vi "Shift Tag offsets for newly inserted data.vi"(4 "Litt/BigEnd":bool, 5 "Amount of data added\n(<0 means # of data bytesremoved)":i32, 6 "Ignore Tags":u16[](array[numeric]), 7 "error in":errorcluster, 8 "Byte stream offset\nwhere new data added":u32, 9 "Directories":T1[](array[typedef]), 10 "Image Data":u8[](array[numeric])) -> (0 "error out":errorcluster, 2 "Directories out":T1[](array[typedef]), 3 "Image Data Out":u8[](array[numeric]))   [LabVIEW 2013, in "Tiff reader.lvlib"]
doc: "This .vi shifts the tag Offsets for newly inserted data that might be inserted before the tags. or their pointer locations."
uses:
  Tiff reader.lvlib
  IFD Entry.ctl
  FieldTypes.ctl
  Word to bytes.vi
  Long word to bytes.vi
  Bytes to long word.vi
panel:
  out "Shifted?":bool
  out "Cluster":T1
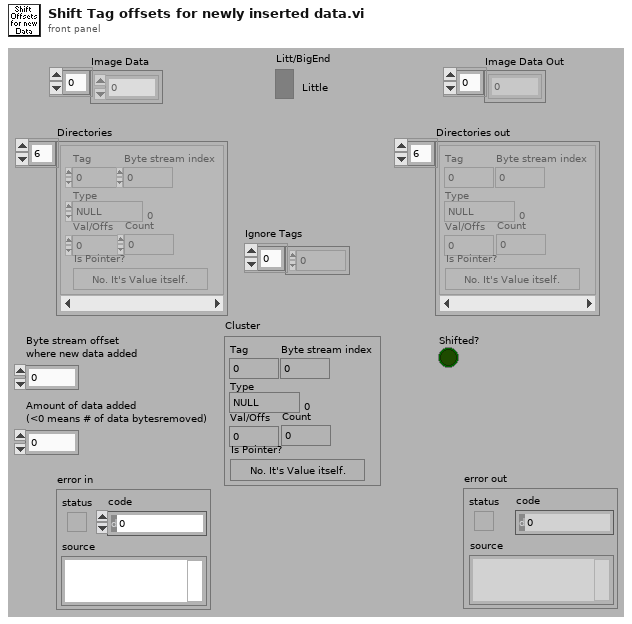
[diagram p1: front panel]
types:
  T1 = typedef "Tiff reader.lvlib/IFD Entry.ctl" = cluster{"Tag":u16, "Type":T2, "Count":u32, "Val/Offs":u32, "Is Pointer?":bool, "Byte stream index":i32}
  T2 = typedef "Tiff reader.lvlib/FieldTypes.ctl" = enum16{"NULL", "U8", "ASCII7", "U16", "U32", "RATIONAL", "SByte(I8)", "Undef(8Bit)", "I16", "I32", "SRat(4B:4B)", "SGL(4Byte)", "DBL(8Byte)"}
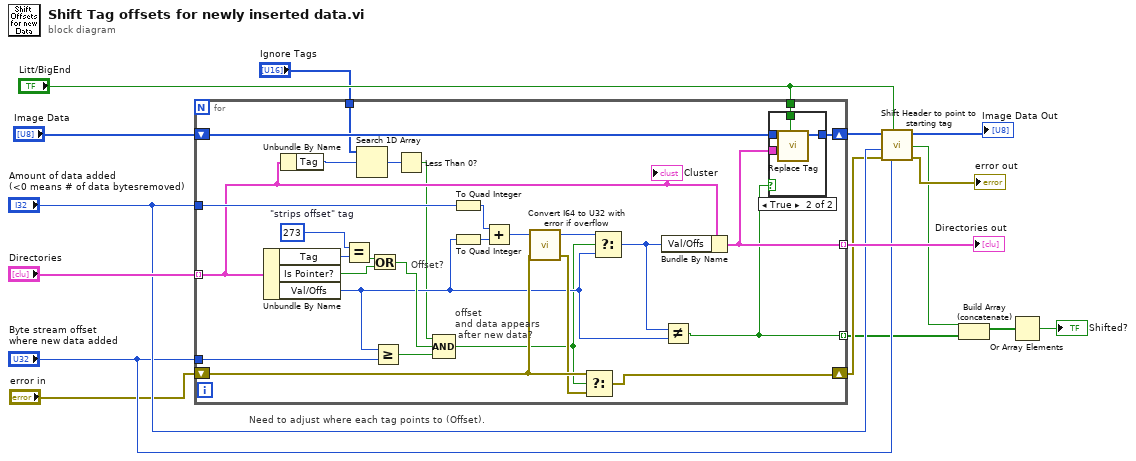
[diagram p0: block diagram]
diagram:
  # "Need to adjust where each tag points to (Offset)."
  n1 = for {
    tunnel: "Directories" -> [w20] mode=indexing
    tunnel: "Byte stream offset\nwhere new data added" -> [w42]
    tunnel: [w34] -> w15 mode=indexing
    tunnel: "Amount of data added\n(<0 means # of data bytesremoved)" -> [w39]
    tunnel: "Litt/BigEnd" -> [w37]
    shift-right: [w35] -> w13
    shift-left: "Image Data" -> [w36]
    shift-right: [w22] -> w8
    shift-left: "error in" -> [w44]
    tunnel: [w24] -> w4 mode=indexing
    tunnel: "Ignore Tags" -> [w21]
    w32 = u16 273  # "strips offset" tag
    # "Offset?"
    # "offset\nand data appears\n after new data?"
    n2 = Unbundle By Name(w20) -> ("Tag"=w33:u16, "Is Pointer?"=w30:bool, "Val/Offs"=w25:u32)
    n3 = Unbundle By Name(w20) -> ("Tag"=w19:u16)
    n4 = Equal?(x=w32, y=w33) -> (x = y?=w31:bool)
    n5 = Search 1D Array(1D array=w21, element=w19) -> (index of element=w18:i32)  [unwired: 1 in]
    n6 = Or(x=w31, y=w30) -> (x .or. y?=w29:bool)
    n7 = Greater Or Equal?(x=w25, y=w42) -> (x >= y?=w41:bool)
    n8 = Less Than 0?(x=w18) -> (x < 0?=w17:bool)
    n9 = Compound Arithmetic op=AND(w17, w29, w41) -> (w23:bool)
    n10 = To Quad Integer(1:w39) -> (0:w38:i64)
    n11 = To Quad Integer(1:w25) -> (0:w40:i64)
    n12 = Add(x=w38, y=w40) -> (x+y=w28:i64)
    n13 = call "Convert I64 to U32 with error if overflow.vi"("error in"=w44, "I64"=w28) -> ("error out"=w43:errorcluster, "U32"=w27:u32)  [unwired: 2 out]
    n14 = Select(t=w44, s=w23, f=w43) -> (s? t:f=w22:errorcluster)
    n15 = Select(t=w27, s=w23, f=w25) -> (s? t:f=w26:u32)
    n16 = Bundle By Name(cluster=w20, "Val/Offs"=w26) -> (w34:T1)
    n17 = Not Equal?(x=w26, y=w25) -> (x != y?=w24:bool)
    n18 = case shown="True" w24 {
      tunnel: w37 -> [_ w49]
      tunnel: w36 -> [w45 w48]
      tunnel: [w45 w47] -> w35
      tunnel: w34 -> [_ w46]
      frame False {
      }
      frame True {
        n19 = call "Replace Tag.vi"("Litt/BigEnd"=w49, "Tag"=w46, "Image Data in"=w48) -> ("Image Data Out"=w47:u8[])  [unwired: 5 out]
      }
    }
    "Cluster" <- w20
  }
  "Directories out" <- w15
  n20 = call "Shift Header to point to starting tag.vi"("Byte stream offset\ninsertion point where \nnew data/tag added"="Byte stream offset\nwhere new data added", "Litt/BigEnd"="Litt/BigEnd", "error in"=w8, "# bytes added\n(<0 means removed)"="Amount of data added\n(<0 means # of data bytesremoved)", "Image Data"=w13) -> ("error out"=→"error out":errorcluster, "Shifted?"=w3:bool, "Image Data Out"=→"Image Data Out":u8[])  [unwired: 3 in, 1 out]
  n21 = Build Array (concatenate)(w3, w4) -> (w5:bool[])
  n22 = Or Array Elements(Boolean array=w5) -> (logical OR=→"Shifted?":bool)
